vi "Untitled 4.vi"() -> ()   [LabVIEW 2017]
panel:
  out "Numeric":dbl
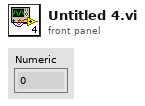
[diagram p1: front panel]
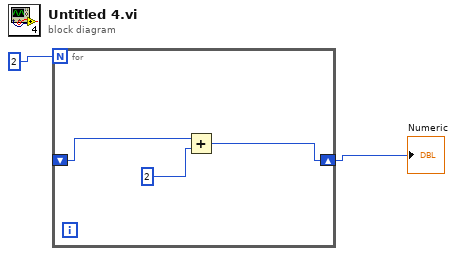
[diagram p0: block diagram]
diagram:
  n1 = for {
    N: 2 -> [_]
    shift-right: [w3] -> w1
    shift-left: _ -> [w5]
    n2 = Add(x=w5, y=2) -> (x+y=w3:i32)
  }
  "Numeric" <- w1
